vi "Debug Sender.vi"   [LabVIEW 2009]
uses:
  TypeDefs/State Machine/Debug Sender States.ctl
  <vilib>/Platform/TimedLoop/XDataNode/XDataNode.xnode
  <vilib>/Platform/TimedLoop/XDataNode/loadlvalarms.vi
  <vilib>/Platform/TimedLoop/XDataNode/timing_clust.ctl
  <vilib>/Platform/TimedLoop/XDataNode/nitl_modes.ctl
  <vilib>/Platform/TimedLoop/XDataNode/wakeup.ctl
  UI Comm/Watchdog Dish Labels.ctl
  <vilib>/Platform/TimedLoop/XDataNode/XDNodeRunTimeDep.lvlib
types:
  T1 = typedef "Debug Sender States.ctl" = enum16{"Check for User", "Send Debug Data"}
  T2 = typedef "UDP Base.ctl" = cluster{"UDP Session":refnum<k16>, "UDP Socket Params":T3}
  T3 = typedef "UDP Socket Params.ctl" = cluster{"Local Port":u16, "Read Timeout":i32, "Write Timeout":i32}
  T4 = typedef "XDNodeRunTimeDep.lvlib/timing_clust.ctl" = cluster{"Expected End [f-1]":u64, "Actual End [f-1]":u64, "Finished Late? [f-1]":bool, "Expected End [i-1]":u64, "Actual End [i-1]":u64, "Finished Late? [i-1]":bool, "Expected Start [i]":u64, "Actual Start [i]":u64, "Expected Start [f]":u64, "Actual Start [f]":u64, "Source Name":string, "Structure Name":string, "Period":i64, "Deadline":i64, "Offset":i64, "Start":i64, "Priority":i32, "Timeout":i32, "Mode":T5, "Wakeup Reason":T6, "Error":errorcluster, "Source Type":string, "Secondary Source Type":string, "Global End Time":u64, "Global Start Time":u64, "Frame Duration":u64, "Iteration Duration":u64, "Assigned CPU":i32, "I/O Scan Engine Mode":u32}
  T5 = typedef "XDNodeRunTimeDep.lvlib/nitl_modes.ctl" = enum32{"No Change", "Process missed periods, maintain original phase", "Discard missed periods, maintain original phase", "Process missed periods, ignore original phase", "Discard missed periods, ignore original phase"}
  T6 = typedef "XDNodeRunTimeDep.lvlib/wakeup.ctl" = enum32{"Normal", "Aborted", "Asynchronous wakeup", "Timing source error", "Timed loop error", "Timeout"}
  T7 = typedef "Watchdog Dish Labels.ctl" = enum16{"GPS", "SICK", "Compass", "Cameras", "Motor Controller", "Debug", "RC Receiver"}
  T8 = typedef "UDP Network Location.ctl" = cluster{"IP Address":string, "Port":u16}
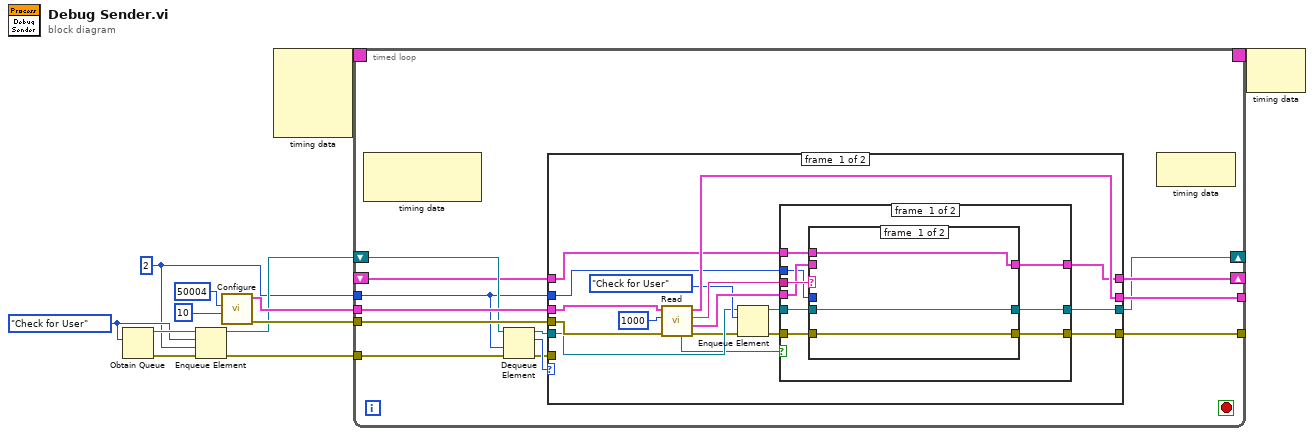
[diagram p0: block diagram]
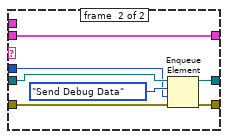
[diagram p2: hidden frame]
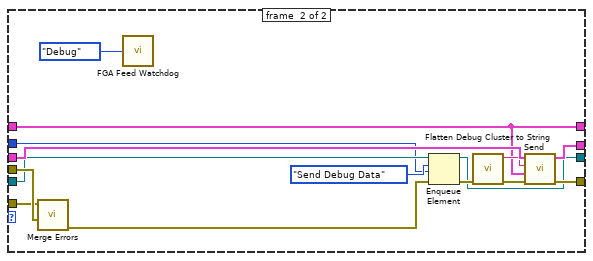
[diagram p4: hidden frame]
diagram:
  w1 = 2 ("timeout in ms (-1)")
  w5 = Debug_Sender_States."Check for User" ("State")
  n1 = Obtain Queue(element data type=w5) -> (queue out=w7:refnum<queue>, error out=w6:errorcluster)  [unwired: 4 in, 1 out]
  n2 = Enqueue Element(queue=w7, element=w5, timeout in ms (-1)=w1, error in (no error)=w6) -> (queue out=w4:refnum<queue>, error out=w3:errorcluster)  [unwired: 1 out]
  n3 = call "Configure.vi"("Read Timeout"=10, "Local Port"=u16 50004) -> ("error out"=w10:errorcluster, "UDP Base out"=w9:T2)  [unwired: 8 in]
  n4 = node-c288() -> (w12:T4)  [unwired: 4 in]
  n5 = timed-loop {
    timing: w12 -> [_]
    timing-out: [_] -> w11
    tunnel: w10 -> [w22]
    tunnel: w9 -> [w25]
    tunnel: [w24] -> _
    tunnel: [w23] -> _
    tunnel: w3 -> [w20]
    shift-right: [w16] -> _
    shift-left: _ -> [w15]
    shift-right: [w14] -> _
    shift-left: w4 -> [w21]
    tunnel: w1 -> [w13]
    stop <- _ stop-if-true
    n6 = node-c288() -> ()  [unwired: 1 in, 2 out]
    n7 = Dequeue Element(queue=w21, timeout in ms (-1)=w13, error in (no error)=w20) -> (queue out=w18:refnum<queue>, element=w19:T1, error out=w17:errorcluster)  [unwired: 1 out]
    n8 = case shown="\"Send Debug Data\"" w19 {
      tunnel: w25 -> [w42 w73]
      tunnel: [w39 w79] -> w24
      tunnel: [w29 w78] -> w23
      tunnel: w22 -> [w41 w77]
      tunnel: w18 -> [w35 w69]
      tunnel: w17 -> [_ w76]
      tunnel: [w37 w67] -> w16
      tunnel: w15 -> [w33 w67]
      tunnel: [w30 w68] -> w14
      tunnel: w13 -> [w27 w66]
      frame #0 {
        n9 = call "Read.vi"("error in (no error)"=w41, "max size (548)"=1000, "UDP Base in"=w42) -> ("error out"=w34:errorcluster, "Network Location"=w38:T8, "Receive Data"=w40:string, "UDP Base out"=w39:T2, "Timeout"=w28:bool)  [unwired: 3 in, 1 out]
        n10 = Enqueue Element(queue=w35, element=Debug_Sender_States."Check for User" ("State"), error in (no error)=w34) -> (queue out=w32:refnum<queue>, error out=w31:errorcluster)  [unwired: 1 in, 1 out]
        n11 = case shown="False" w28 {
          tunnel: w40 -> [w51 _]
          tunnel: w38 -> [w50 _]
          tunnel: [w49 w62] -> w37
          tunnel: w33 -> [w48 w62]
          tunnel: w32 -> [w47 w64]
          tunnel: w31 -> [w46 w63]
          tunnel: [w45 w64] -> w30
          tunnel: [w44 w63] -> w29
          tunnel: w27 -> [w43 _]
          frame #0 {
            n12 = case shown="\"Q-DATA-REQUEST\"" w51 {
              tunnel: w50 -> [_ w61]
              tunnel: [w54 w61] -> w49
              tunnel: w48 -> [w54 _]
              tunnel: w47 -> [w53 w60]
              tunnel: w46 -> [w52 w59]
              tunnel: [w53 w58] -> w45
              tunnel: [w52 w57] -> w44
              tunnel: w43 -> [_ w55]
              frame #0 {
              }
              frame #1 {
                n13 = Enqueue Element(queue=w60, element=Debug_Sender_States."Send Debug Data", timeout in ms (-1)=w55, error in (no error)=w59) -> (queue out=w58:refnum<queue>, error out=w57:errorcluster)  [unwired: 1 out]
              }
            }
          }
          frame #1 {
          }
        }
      }
      frame #1 {
        n14 = call <vilib>:"Merge Errors.vi"("error in 3 (no error)"=w77, "error in 1 (no error)"=w76) -> ("error out"=w74:errorcluster)  [unwired: 5 in]
        n15 = call "FGA Feed Watchdog.vi"("Watchdog Dish"=Watchdog_Dish_Labels."Debug") -> ()  [unwired: 1 out]
        n16 = Enqueue Element(queue=w69, element=Debug_Sender_States."Send Debug Data" ("State"), timeout in ms (-1)=w66, error in (no error)=w74) -> (queue out=w68:refnum<queue>, error out=w72:errorcluster)  [unwired: 1 out]
        n17 = call "Flatten Debug Cluster to String.vi"("error in (no error)"=w72) -> ("error out"=w71:errorcluster, "Flattened Cluster"=w70:string)  [unwired: 9 in]
        n18 = call "Send.vi"("error in (no error)"=w71, "Destination Location"=w67, "Send Data"=w70, "UDP Base in"=w73) -> ("error out"=w78:errorcluster, "UDP Base out"=w79:T2)  [unwired: 5 in, 1 out]
      }
    }
    n19 = node-c288() -> ()  [unwired: 1 in, 1 out]
  }
  n20 = node-c288(w11) -> ()  [unwired: 1 out]
